vi "Insert Error if occured (SubVI).vi"(8 "error in (no error)":errorcluster, 10 "Error messages":string[](array[string]), 11 "Error conditionals":bool[](array[boolean])) -> (0 "error out":errorcluster)   [LabVIEW 2009, in "MicroDAQ.lvlib"]
uses:
  <instrlib>/MicroDAQ/MicroDAQ.lvlib
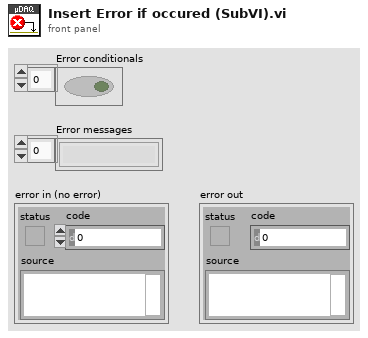
[diagram p1: front panel]
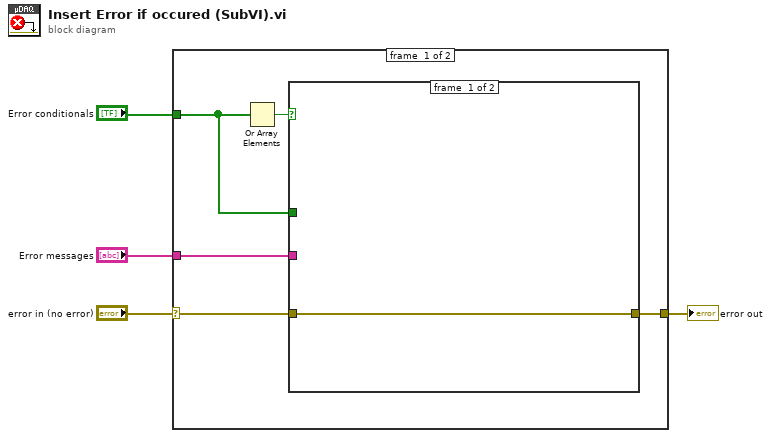
[diagram p0: block diagram]
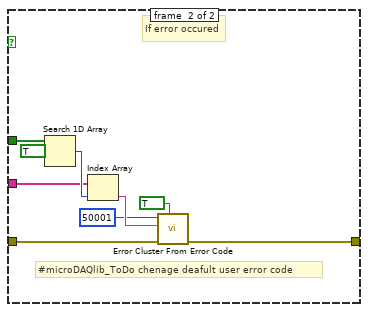
[diagram p2: hidden frame]
diagram:
  n1 = case shown="No Error" "error in (no error)" {
    selector: "error in (no error)" -> [w6 w20]
    tunnel: "Error messages" -> [w9 _]
    tunnel: "Error conditionals" -> [w8 _]
    tunnel: [w5 w20] -> w1
    frame #0 {
      n2 = Or Array Elements(Boolean array=w8) -> (logical OR=w7:bool)
      n3 = case shown="True" w7 {
        tunnel: [w10 w19] -> w5
        tunnel: w6 -> [w10 w18]
        tunnel: w8 -> [_ w17]
        tunnel: w9 -> [_ w14]
        frame #0 {
        }
        frame #1 {
          # "#microDAQlib_ToDo chenage deafult user error code"
          # "If error occured"
          n4 = Search 1D Array(1D array=w17, element=TRUE) -> (index of element=w15:i32)  [unwired: 1 in]
          n5 = Index Array(array=w14, index=w15) -> (element=w13:string)
          n6 = call <vilib>:"Error Cluster From Error Code.vi"("show call chain? (False)"=TRUE, "error in (no error)"=w18, "error message (\"\")"=w13, "error code (0)"=50001) -> ("error out"=w19:errorcluster)  [unwired: 5 in]
        }
      }
    }
    frame #1 {
    }
  }
  "error out" <- w1
